vi "Detect Single (Greyscale).vi"(8 "error in (no error)":errorcluster, 10 "Greyscale Image in":T1, 11 "QR Code Detector in":refnum<class "QR Code Detector.lvclass">) -> (0 "error out":errorcluster, 1 "Detection":T2, 2 "Greyscale Image":T1, 3 "QR Code Detector":refnum<class "QR Code Detector.lvclass">, 4 "Detected":bool)   [LabVIEW 2020, in "feature_detection.lvlib" / "QR Code Detector.lvclass"]
doc: "Detect a single QR Code in an Image. If multiple QR Codes are present then only one detection will be returned."
uses:
  QR Code Detector.lvclass
  image/Greyscale Image.ctl
  common/Image Points Quad (Float).ctl
  common/Image Point (Float).ctl
  QR Code Detector.lvclass/QR Code Detector.ctl
  3f237dad-095a-4622-b7ca-85271485a49f.vi
  <vilib>/Utility/error.llb/Error Cluster From Error Code.vi
  common/common.lvlib
  image/image.lvlib
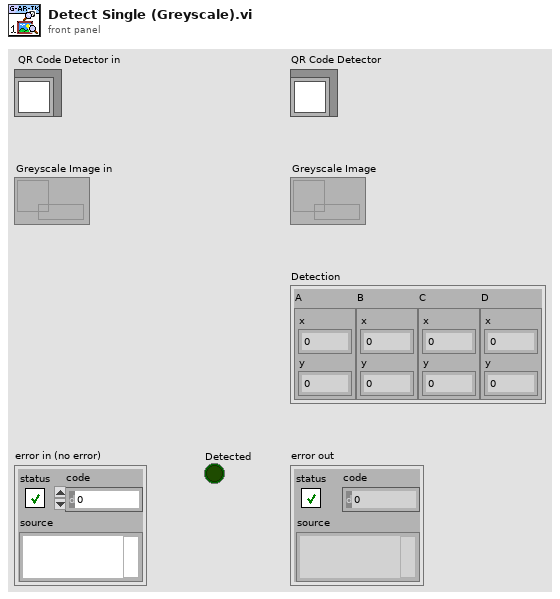
[diagram p1: front panel]
types:
  T1 = typedef "image.lvlib/Greyscale Image.ctl" = refnum<data-value>
  T2 = typedef "common.lvlib/Image Points Quad (Float).ctl" = cluster{"A":T3, "B":T3, "C":T3, "D":T3}
  T3 = typedef "common.lvlib/Image Point (Float).ctl" = cluster{"x":dbl, "y":dbl}
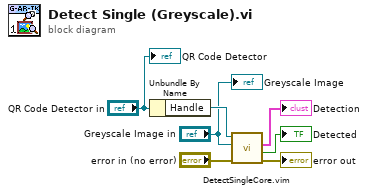
[diagram p0: block diagram]
diagram:
  n1 = Unbundle By Name("QR Code Detector in") -> ("Handle"=w5:refnum<data-value>)
  n2 = call "DetectSingleCore.vim"("error in (no error)"="error in (no error)", "Greyscale Image"="Greyscale Image in", "Handle"=w5) -> ("error out"=→"error out":errorcluster, "Detected"=→"Detected":bool, "Detection"=→"Detection":T2)  [unwired: 6 in]
  "QR Code Detector" <- "QR Code Detector in"
  "Greyscale Image" <- "Greyscale Image in"
